vi "send_data_ack (SubVI).vi"(4 "command":i32, 5 "number data":i32=1, 6 "adreça":i32, 7 "Dada":i32, 8 "error out":errorcluster, 9 "Send":bool, 10 "id":i32, 11 "connection ID":refnum<k5>) -> (0 "error out 2":errorcluster, 1 "bytes written":i32, 2 "data out":string, 3 "connection ID out":refnum<k5>)   [LabVIEW 2009]
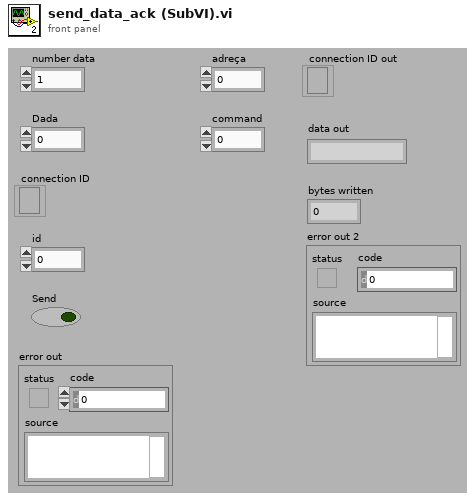
[diagram p1: front panel]
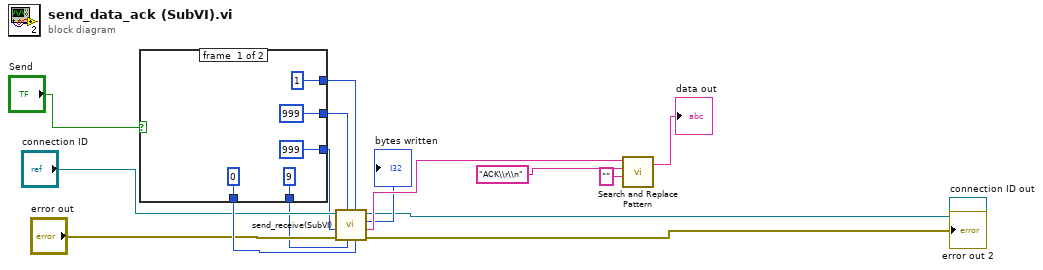
[diagram p0: block diagram]
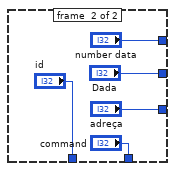
[diagram p2: hidden frame]
diagram:
  n1 = case shown="True" "Send" {
    tunnel: [999 ("adreça") "adreça"] -> w2
    tunnel: [9 ("command") "command"] -> w3
    tunnel: [999 ("Dada") "Dada"] -> w4
    tunnel: [1 ("number data") "number data"] -> w5
    tunnel: [0 ("id") "id"] -> w10
    frame #0 {
    }
    frame #1 {
    }
  }
  n2 = call "send_receive(SubVI).vi"("id"=w10, "number data"=w5, "Action"=w3, "Data"=w4, "error in"="error out", "Address"=w2, "connection ID"="connection ID") -> ("error out"=→"error out 2":errorcluster, "data out"=w13:string, "bytes written"=→"bytes written":i32, "connection ID out"=→"connection ID out":refnum<k5>)  [unwired: 1 in]
  n3 = call <vilib>:"Search and Replace Pattern.vi"("string"=w13, "regular expression (\"\")"="ACK\\r\\n" ("regular expression (\"\")"), "replace string (\"\")"="" ("replace string (\"\")")) -> ("result string"=→"data out":string)  [unwired: 2 in, 1 out]
